vi "One_Tote_Fault_Detection.vi"(11 "1_Tote_Enable":bool=TRUE) -> ()   [LabVIEW 2014]
uses:
  General_VI/Global Var.vi
panel:
  in  "Time _To_Drive_1_Tote":i32=8000
  in  "Extend_Flipper_Time":i32=500
  in  "Open_Infeed_time":i32=800
  # "Static Tunning Values"
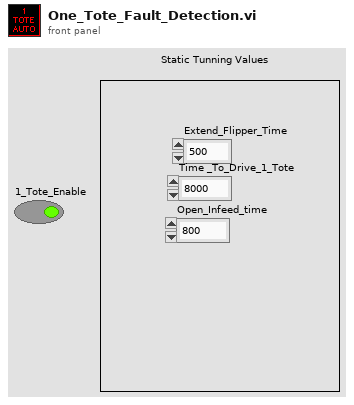
[diagram p1: front panel]
types:
  T1 = cluster{"Open_Infeed_time":i32, "Extend_Flipper_Time":i32, "Time _To_Drive_1_Tote":i32}
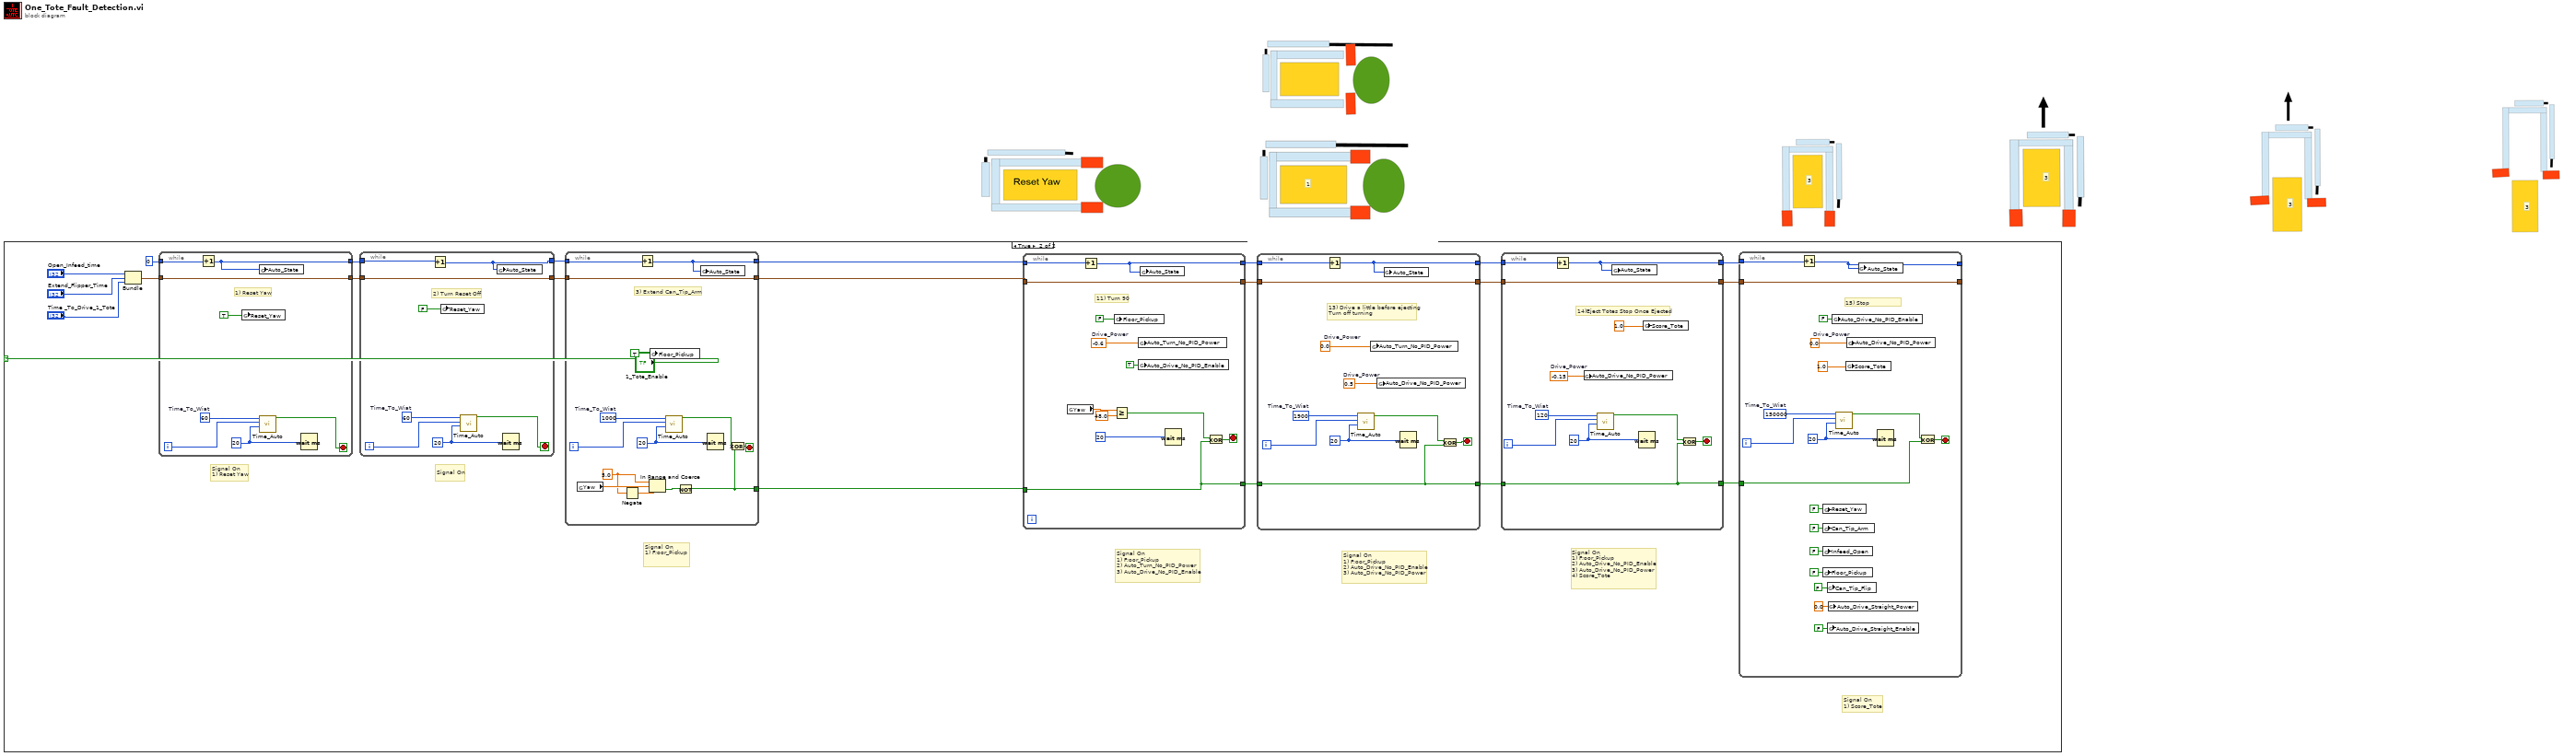
[diagram p0: block diagram]
diagram:
  # "3"
  # "3"
  # "3"
  # "3"
  # "1"
  n1 = case shown="True" "1_Tote_Enable" {
    frame False {
    }
    frame True {
      # "Signal On\n1) Score_Tote"
      # "Signal On\n1) F;oor_Pickup\n2) Auto_Drive_No_PID_Enable\n3) Auto_Drive_No_PID_Power\n4) Score_Tote"
      # "Signal On\n1) F;oor_Pickup\n2) Auto_Drive_No_PID_Enable\n3) Auto_Drive_No_PID_Power"
      # "Signal On\n1) F;oor_Pickup\n2) Auto_Turn_No_PID_Power\n3) Auto_Drive_No_PID_Enable"
      # "Signal On\n1) F;oor_Pickup"
      # "Signal On"
      # "Signal On\n1) Reset Yaw"
      n2 = Bundle("Open_Infeed_time"="Open_Infeed_time", "Extend_Flipper_Time"="Extend_Flipper_Time", "Time _To_Drive_1_Tote"="Time _To_Drive_1_Tote") -> (w15:T1)  [unwired: 1 in]
      n3 = while {
        tunnel: 0 -> [w99]
        tunnel: [w98] -> w21
        tunnel: w15 -> [w100]
        tunnel: [w100] -> w14
        i -> [w103]
        stop <- w105 stop-if-true
        w104 = u32 20 ("milliseconds to wait")
        w102 = 60  # Time_To_Wiat
        # "1) Reset Yaw"
        n4 = Increment(x=w99) -> (x+1=w98:i32)
        n5 = global write "Global Var.vi" "Reset_Yaw"(TRUE) -> ()
        n6 = global write "Global Var.vi" "Auto_State"(w98) -> ()
        n7 = call "Time_Auto.vi"("Sample_Time"=w104, "Counter"=w103, "Time_to_wait"=w102) -> ("Boolean"=w105:bool)  [unwired: 8 in]
        n8 = Wait (ms)(milliseconds to wait=w104) -> ()  [unwired: 1 out]
      }
      n9 = while {
        tunnel: w21 -> [w91]
        tunnel: [w90] -> w20
        tunnel: w14 -> [w92]
        tunnel: [w92] -> w13
        i -> [w95]
        stop <- w97 stop-if-true
        w96 = u32 20 ("milliseconds to wait")
        w94 = 60  # Time_To_Wiat
        # "2) Turn Reset Off"
        n10 = Increment(x=w91) -> (x+1=w90:i32)
        n11 = global write "Global Var.vi" "Reset_Yaw"(FALSE) -> ()
        n12 = call "Time_Auto.vi"("Sample_Time"=w96, "Counter"=w95, "Time_to_wait"=w94) -> ("Boolean"=w97:bool)  [unwired: 8 in]
        n13 = global write "Global Var.vi" "Auto_State"(w90) -> ()
        n14 = Wait (ms)(milliseconds to wait=w96) -> ()  [unwired: 1 out]
      }
      n15 = while {
        tunnel: w20 -> [w85]
        tunnel: [w84] -> w6
        tunnel: w13 -> [w86]
        tunnel: [w86] -> w5
        tunnel: [w76] -> w4
        i -> [w88]
        stop <- w78 stop-if-true
        w80 = 5.0 ("upper limit")
        w89 = u32 20 ("milliseconds to wait")
        w87 = 1000  # Time_To_Wiat
        # "3) Extend Can_Tip_Arm"
        n16 = global read "Global Var.vi" "Yaw"() -> (w82:dbl)
        n17 = Negate(x=w80) -> (-x=w81:dbl)
        n18 = Increment(x=w85) -> (x+1=w84:i32)
        n19 = In Range and Coerce(upper limit=w80, x=w82, lower limit=w81) -> (In Range?=w77:bool)  [unwired: 1 out]
        n20 = global write "Global Var.vi" "Floor_Pickup"(TRUE) -> ()
        n21 = call "Time_Auto.vi"("Sample_Time"=w89, "Counter"=w88, "Time_to_wait"=w87) -> ("Boolean"=w79:bool)  [unwired: 8 in]
        n22 = Not(x=w77) -> (.not. x?=w76:bool)
        n23 = global write "Global Var.vi" "Auto_State"(w84) -> ()
        n24 = Wait (ms)(milliseconds to wait=w89) -> ()  [unwired: 1 out]
        n25 = Exclusive Or(1:w76, 2:w79) -> (0:w78:bool)
      }
      n26 = while {
        tunnel: w6 -> [w70]
        tunnel: [w69] -> w19
        tunnel: w5 -> [w71]
        tunnel: [w71] -> w12
        tunnel: w4 -> [w64]
        tunnel: [w64] -> w9
        stop <- w66 stop-if-true
        w68 = -0.6  # Drive_Power
        # "11) Turn 90"
        n27 = global read "Global Var.vi" "Yaw"() -> (w73:dbl)
        n28 = Increment(x=w70) -> (x+1=w69:i32)
        n29 = Greater Or Equal?(x=w73, y=48.0) -> (x >= y?=w65:bool)
        n30 = global write "Global Var.vi" "Floor_Pickup"(FALSE) -> ()
        n31 = global write "Global Var.vi" "Auto_Turn_No_PID_Power"(w68) -> ()
        n32 = global write "Global Var.vi" "Auto_Drive_No_PID_Enable"(TRUE ("Auto_Drive_No_PID_Enable")) -> ()
        n33 = global write "Global Var.vi" "Auto_State"(w69) -> ()
        n34 = Wait (ms)(milliseconds to wait=u32 20) -> ()  [unwired: 1 out]
        n35 = Exclusive Or(1:w64, 2:w65) -> (0:w66:bool)
      }
      n36 = while {
        tunnel: w19 -> [w58]
        tunnel: [w57] -> w2
        tunnel: w12 -> [w59]
        tunnel: [w59] -> w11
        tunnel: w9 -> [w53]
        tunnel: [w53] -> w8
        i -> [w62]
        stop <- w55 stop-if-true
        w56 = 0.0  # Drive_Power
        w60 = 0.5  # Drive_Power
        w63 = u32 20 ("milliseconds to wait")
        w61 = 1900  # Time_To_Wiat
        # "13) Drive a little before ejecting\nTurn off turning"
        n37 = Increment(x=w58) -> (x+1=w57:i32)
        n38 = call "Time_Auto.vi"("Sample_Time"=w63, "Counter"=w62, "Time_to_wait"=w61) -> ("Boolean"=w54:bool)  [unwired: 8 in]
        n39 = global write "Global Var.vi" "Auto_Turn_No_PID_Power"(w56) -> ()
        n40 = global write "Global Var.vi" "Auto_Drive_No_PID_Power"(w60) -> ()
        n41 = global write "Global Var.vi" "Auto_State"(w57) -> ()
        n42 = Wait (ms)(milliseconds to wait=w63) -> ()  [unwired: 1 out]
        n43 = Exclusive Or(1:w53, 2:w54) -> (0:w55:bool)
      }
      n44 = while {
        tunnel: w2 -> [w47]
        tunnel: [w46] -> w3
        tunnel: w11 -> [w48]
        tunnel: [w48] -> w10
        tunnel: w8 -> [w42]
        tunnel: [w42] -> w7
        i -> [w51]
        stop <- w44 stop-if-true
        w45 = -0.15  # Drive_Power
        w52 = u32 20 ("milliseconds to wait")
        w50 = 120  # Time_To_Wiat
        # "14)Eject Totes Stop Once Ejected"
        n45 = Increment(x=w47) -> (x+1=w46:i32)
        n46 = global write "Global Var.vi" "Auto_Drive_No_PID_Power"(w45) -> ()
        n47 = call "Time_Auto.vi"("Sample_Time"=w52, "Counter"=w51, "Time_to_wait"=w50) -> ("Boolean"=w43:bool)  [unwired: 8 in]
        n48 = global write "Global Var.vi" "Auto_State"(w46) -> ()
        n49 = Wait (ms)(milliseconds to wait=w52) -> ()  [unwired: 1 out]
        n50 = global write "Global Var.vi" "Score_Tote"(1.0) -> ()
        n51 = Exclusive Or(1:w42, 2:w43) -> (0:w44:bool)
      }
      n52 = while {
        tunnel: w3 -> [w36]
        tunnel: w10 -> [w37]
        tunnel: [w37] -> _
        tunnel: [w35] -> _
        tunnel: w7 -> [w30]
        i -> [w40]
        stop <- w32 stop-if-true
        w33 = 0.0  # Drive_Power
        w41 = u32 20 ("milliseconds to wait")
        w39 = 150000  # Time_To_Wiat
        # "15) Stop"
        n53 = Increment(x=w36) -> (x+1=w35:i32)
        n54 = global write "Global Var.vi" "Reset_Yaw"(FALSE ("Reset_Yaw")) -> ()
        n55 = global write "Global Var.vi" "Can_Tip_Arm"(FALSE ("Can_Tip_Arm")) -> ()
        n56 = global write "Global Var.vi" "Infeed_Open"(FALSE ("Infeed_Open")) -> ()
        n57 = global write "Global Var.vi" "Floor_Pickup"(FALSE ("Floor_Pickup")) -> ()
        n58 = global write "Global Var.vi" "Can_Tip_Flip"(FALSE ("Can_Tip_Flip")) -> ()
        n59 = global write "Global Var.vi" "Auto_Drive_Straight_Enable"(FALSE ("Auto_Drive_Straight_Enable")) -> ()
        n60 = global write "Global Var.vi" "Auto_Drive_Straight_Power"(0.0 ("Auto_Drive_Straight_Power")) -> ()
        n61 = global write "Global Var.vi" "Auto_Drive_No_PID_Enable"(FALSE ("Auto_Drive_No_PID_Enable")) -> ()
        n62 = call "Time_Auto.vi"("Sample_Time"=w41, "Counter"=w40, "Time_to_wait"=w39) -> ("Boolean"=w31:bool)  [unwired: 8 in]
        n63 = global write "Global Var.vi" "Score_Tote"(1.0) -> ()
        n64 = global write "Global Var.vi" "Auto_Drive_No_PID_Power"(w33) -> ()
        n65 = global write "Global Var.vi" "Auto_State"(w35) -> ()
        n66 = Wait (ms)(milliseconds to wait=w41) -> ()  [unwired: 1 out]
        n67 = Exclusive Or(1:w30, 2:w31) -> (0:w32:bool)
      }
    }
  }
